vi "Get Variables.vi"(8 "error in (no error)":errorcluster, 11 "Message Popup in":refnum<class "Generate Random Data.lvclass">) -> (0 "error out":errorcluster, 2 "Variables":variant, 3 "Message Popup out":refnum<class "Generate Random Data.lvclass">)   [LabVIEW 2016, in "Generate Random Data.lvclass"]
uses:
  Generate Random Data.lvclass
  Generate Random Data.lvclass/Generate Random Data.ctl
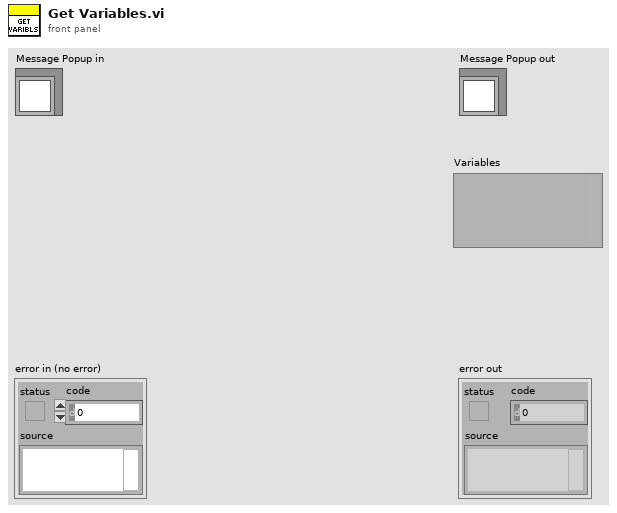
[diagram p1: front panel]
types:
  T1 = typedef "Generate Random Data.lvclass/Variables.ctl" = cluster{"sample":string}
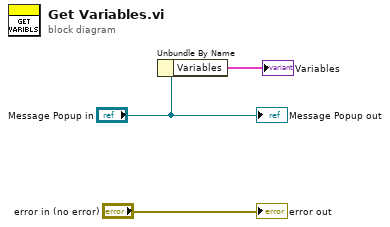
[diagram p0: block diagram]
diagram:
  n1 = Unbundle By Name("Message Popup in") -> ("Variables"=→"Variables":T1)
  "error out" <- "error in (no error)"
  "Message Popup out" <- "Message Popup in"
